vi "Get Harmonic Multiplier.vi"(8 "error in (no error)":errorcluster, 11 "Handle in":i32) -> (0 "error out":errorcluster, 2 "Harmonic Multiplier":i32, 3 "Handle out":i32)   [LabVIEW 2013, in "Thorlabs_MC2000B.lvlib"]
uses:
  <instrlib>/Thorlabs_MC2000B/Thorlabs_MC2000B.lvlib
  <instrlib>/Thorlabs_MC2000B/Library/MC2000CommandLibWin32.dll
  Program Files/National Instruments/LabVIEW 2011/instr.lib/Thorlabs_MC2000B/Library/MC2000CommandLibWin64.dll
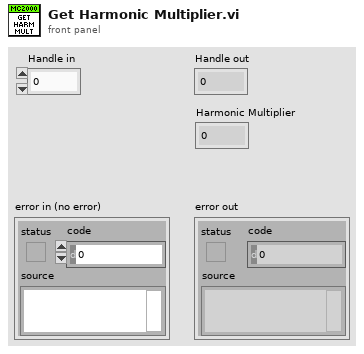
[diagram p1: front panel]
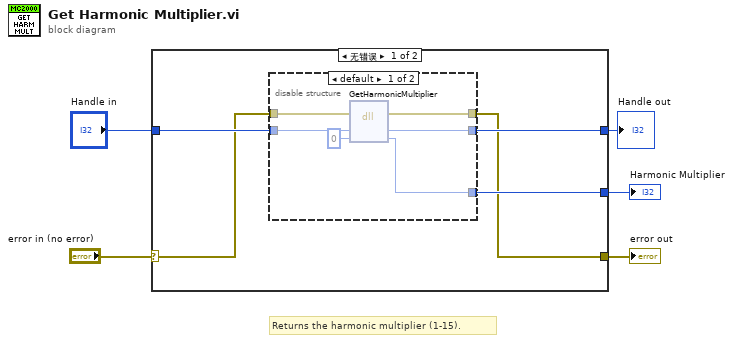
[diagram p0: block diagram]
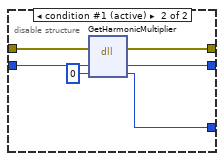
[diagram p2: hidden frame]
diagram:
  # "Returns the harmonic multiplier (1-15)."
  n1 = case shown="无错误" "error in (no error)" {
    selector: "error in (no error)" -> [w6 w24]
    tunnel: [w8 _] -> w5
    tunnel: [w7 w24] -> w4
    tunnel: "Handle in" -> [w10 w23]
    tunnel: [w9 w23] -> w1
    frame No Error {
      n2 = disable-structure shown="default" {
        disable-tunnel: w10 -> [w16 w22]
        disable-tunnel: [w15 w21] -> w9
        disable-tunnel: [w13 w19] -> w8
        disable-tunnel: [w12 w18] -> w7
        disable-tunnel: w6 -> [w11 w17]
        frame condition #0 {
          n3 = dll-call lib="D:/Program Files/National Instruments/LabVIEW 2011/instr.lib/Thorlabs_MC2000B/Library/MC2000CommandLibWin64.dll" fn="GetHarmonicMultiplier"(error in=w11, "hdl"=w16, "nharmonic"=0) -> (error out=w12:errorcluster, "hdl"=w15:i32, "nharmonic"=w13:i32)  [unwired: 3 in, 1 out]
        }
        frame condition #1 (active) {
          n4 = dll-call lib="C:/Program Files (x86)/National Instruments/LabVIEW 2013/instr.lib/Thorlabs_MC2000B/Library/MC2000CommandLibWin32.dll" fn="GetHarmonicMultiplier"(error in=w17, "hdl"=w22, "nharmonic"=0) -> (error out=w18:errorcluster, "hdl"=w21:i32, "nharmonic"=w19:i32)  [unwired: 3 in, 1 out]
        }
      }
    }
    frame Error {
    }
  }
  "error out" <- w4
  "Harmonic Multiplier" <- w5
  "Handle out" <- w1
